vi "number2-globe.vi"() -> ()   [LabVIEW 2014]
panel:
  out "Tilted":cluster{dbl[], dbl[]}(graph)
  out "Original":cluster{dbl[], dbl[]}(graph)
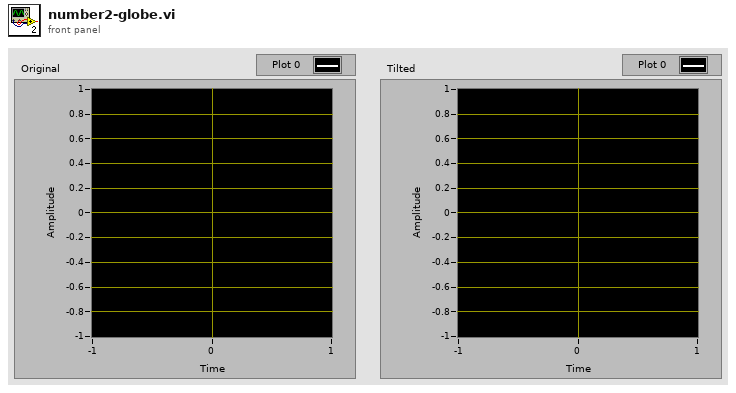
[diagram p1: front panel]
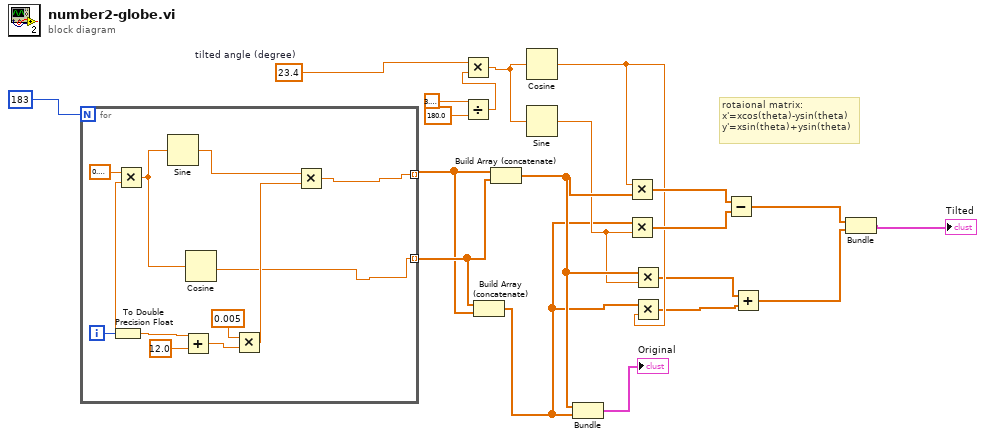
[diagram p0: block diagram]
diagram:
  w1 = 23.4  # tilted angle (degree)
  # "rotaional matrix:\nx'=xcos(theta)-ysin(theta)\ny'=xsin(theta)+ysin(theta)"
  n1 = for {
    N: 183 -> [_]
    tunnel: [w22] -> w19 mode=indexing
    tunnel: [w21] -> w18 mode=indexing
    i -> [w30]
    n2 = To Double Precision Float(number=w30) -> (double precision float=w24:dbl)
    n3 = Multiply(x=0.3183098861837907, y=w24) -> (x*y=w25:dbl)
    n4 = Sine(x=w25) -> (sin(x)=w23:dbl)
    n5 = Add(x=w24, y=12.0) -> (x+y=w28:dbl)
    n6 = Cosine(x=w25) -> (cos(x)=w22:dbl)
    n7 = Multiply(x=0.005, y=w28) -> (x*y=w27:dbl)
    n8 = Multiply(x=w23, y=w27) -> (x*y=w21:dbl)
  }
  n9 = Divide(x=3.141592653589793, y=180.0) -> (x/y=w2:dbl)
  n10 = Multiply(x=w1, y=w2) -> (x*y=w3:dbl)
  n11 = Build Array (concatenate)(w19, w18) -> (w11:dbl[])
  n12 = Build Array (concatenate)(w18, w19) -> (w13:dbl[])
  n13 = Cosine(x=w3) -> (cos(x)=w10:dbl)
  n14 = Sine(x=w3) -> (sin(x)=w12:dbl)
  n15 = Bundle(w13, w11) -> (→"Original":cluster{dbl[], dbl[]})  [unwired: 1 in]
  n16 = Multiply(x=w10, y=w13) -> (x*y=w16:dbl[])
  n17 = Multiply(x=w11, y=w12) -> (x*y=w15:dbl[])
  n18 = Multiply(x=w13, y=w12) -> (x*y=w9:dbl[])
  n19 = Multiply(x=w11, y=w10) -> (x*y=w8:dbl[])
  n20 = Subtract(x=w16, y=w15) -> (x-y=w14:dbl[])
  n21 = Add(x=w9, y=w8) -> (x+y=w7:dbl[])
  n22 = Bundle(w14, w7) -> (→"Tilted":cluster{dbl[], dbl[]})  [unwired: 1 in]
